vi "Day 20-Calculate Infinity Value.vi"(10 "Lookup Array":bool[](array[boolean]), 11 "Previous \"Infinity\" Value":bool) -> (3 "New \"Infinity\" Value":bool)   [LabVIEW 2021]
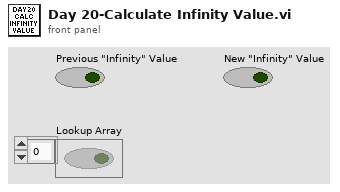
[diagram p1: front panel]
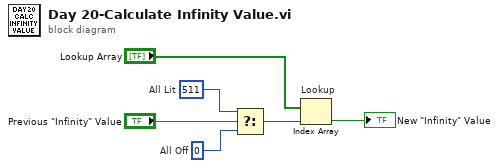
[diagram p0: block diagram]
diagram:
  w2 = 511  # All Lit
  w1 = 0  # All Off
  n1 = Select(t=w2, s="Previous \"Infinity\" Value", f=w1) -> (s? t:f=w3:i32)
  n2 = Index Array "Lookup"(array="Lookup Array", index=w3) -> (element=→"New \"Infinity\" Value":bool)
